vi "BRig_RT_comm_webdav_upload_all__genericSendAll.vi"(0 "input_hSession":T1, 1 "input_arrFilenames":string[](array[string]), 2 "input_n":i32, 5 "input_error":errorcluster, 7 "input_arrUploaded":bool[](array[boolean]), 9 "input_arrSentTarget":bool[](array[boolean]), 11 "input_arrSentTargetSpare":bool[](array[boolean]), 12 "input_fileName_prefix":string, 13 "input_Target(F)_or_Spare(T)":bool) -> (4 "output_hSession":T1, 6 "output_error":errorcluster, 8 "output_arrUploaded":bool[](array[boolean]), 10 "output_arrSentTarget":bool[](array[boolean]), 15 "output_arrSentTargetSpare":bool[](array[boolean]))   [LabVIEW 2014]
uses:
  <vilib>/WebDAVClient/Advanced/SessionHandle.ctl
  <vilib>/WebDAVClient/NI_WebDAV.lvlib
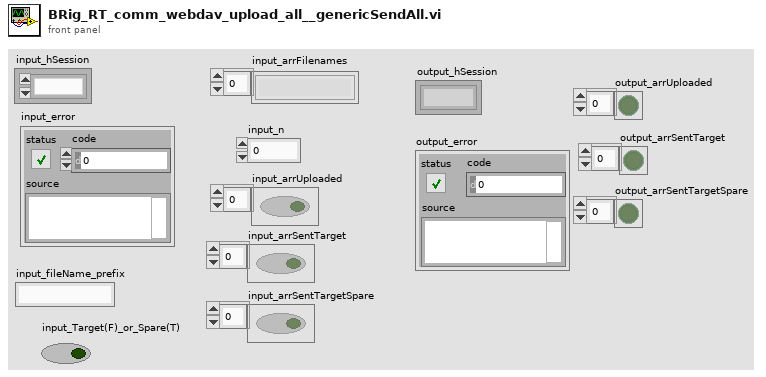
[diagram p1: front panel]
types:
  T1 = typedef "NI_WebDAV.lvlib/SessionHandle.ctl" = refnum<k1>
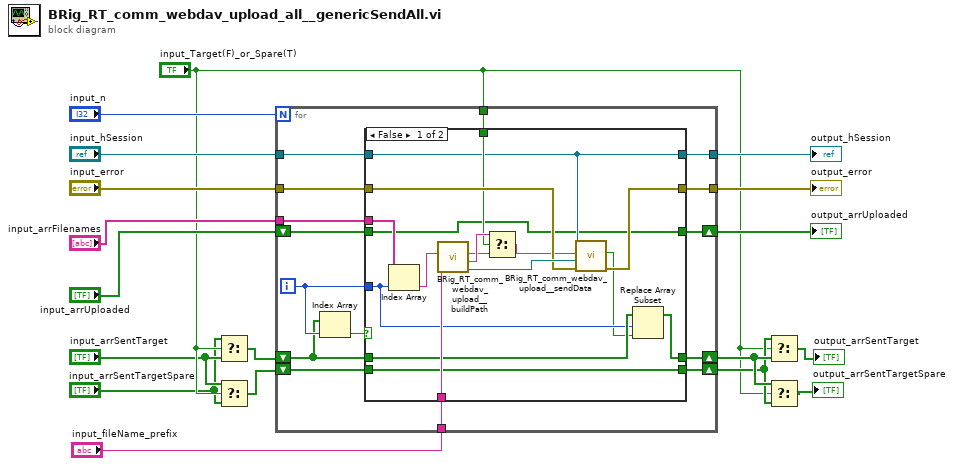
[diagram p0: block diagram]
diagram:
  n1 = Select(t="input_arrSentTargetSpare", s="input_Target(F)_or_Spare(T)", f="input_arrSentTarget") -> (s? t:f=w2:bool[])
  n2 = Select(t="input_arrSentTarget", s="input_Target(F)_or_Spare(T)", f="input_arrSentTargetSpare") -> (s? t:f=w1:bool[])
  n3 = for {
    N: "input_n" -> [_]
    tunnel: "input_arrFilenames" -> [w33]
    shift-right: [w24] -> w10
    shift-left: "input_arrUploaded" -> [w23]
    tunnel: "input_fileName_prefix" -> [w32]
    tunnel: "input_hSession" -> [w30]
    tunnel: [w25] -> w12
    tunnel: "input_error" -> [w31]
    shift-right: [w21] -> w9
    shift-left: w2 -> [w22]
    shift-right: [w19] -> w8
    shift-left: w1 -> [w20]
    tunnel: [w29] -> w11
    tunnel: "input_Target(F)_or_Spare(T)" -> [w28]
    i -> [w27]
    n4 = Index Array(array=w22, index=w27) -> (element=w26:bool)
    n5 = case shown="False" w26 {
      tunnel: w33 -> [w50 _]
      tunnel: w32 -> [w49 _]
      tunnel: w31 -> [w46 w54]
      tunnel: w30 -> [w40 w55]
      tunnel: [w45 w54] -> w29
      tunnel: w28 -> [w41 _]
      tunnel: w27 -> [w37 _]
      tunnel: [w40 w55] -> w25
      tunnel: [w39 w53] -> w24
      tunnel: w23 -> [w39 w53]
      tunnel: w22 -> [w38 w52]
      tunnel: [w35 w52] -> w21
      tunnel: w20 -> [w34 w51]
      tunnel: [w34 w51] -> w19
      frame False {
        n6 = Index Array(array=w50, index=w37) -> (element=w48:string)
        n7 = call "BRig_RT_comm_webdav_upload__buildPath.vi"("input_fileName_prefix"=w49, "input_fileName"=w48) -> ("output_localPath"=w47:path, "output_targetPath_spare"=w44:string, "output_targetPath"=w43:string)  [unwired: 7 in]
        n8 = Select(t=w44, s=w41, f=w43) -> (s? t:f=w42:string)
        n9 = call "BRig_RT_comm_webdav_upload__sendData.vi"("input_error"=w46, "input_localPath"=w47, "input_targetPath"=w42, "input_hSession"=w40) -> ("error out"=w45:errorcluster, "output_sendData"=w36:bool)  [unwired: 5 in, 1 out]
        n10 = Replace Array Subset(array=w38, new element=w36, index=w37) -> (w35:bool[])
      }
      frame True {
      }
    }
  }
  "output_hSession" <- w12
  "output_error" <- w11
  "output_arrUploaded" <- w10
  n11 = Select(t=w8, s="input_Target(F)_or_Spare(T)", f=w9) -> (s? t:f=→"output_arrSentTarget":bool[])
  n12 = Select(t=w9, s="input_Target(F)_or_Spare(T)", f=w8) -> (s? t:f=→"output_arrSentTargetSpare":bool[])
